vi "Fpga-MicroBlaze-Top.vi"() -> ()   [LabVIEW 2017]
uses:
  <vilib>/Platform/TimedLoop/XDataNode/timing_clust.ctl
  <vilib>/Platform/TimedLoop/XDataNode/nitl_modes.ctl
  <vilib>/Platform/TimedLoop/XDataNode/wakeup.ctl
  <vilib>/rvi/Emulation/niFpgaSctlEmulationGetInTimedLoop.vi
  <vilib>/rvi/Emulation/niFpgaEmulationReportErrorSimple.vi
  <vilib>/rvi/Emulation/niFpgaGetClockAttributes.vi
  <vilib>/rvi/Emulation/niFpgaCriticalErrorInLSC.vi
  <vilib>/rvi/eio/common/nirviEmuTemplateMethod_errors.vi
  <vilib>/rvi/interface/RandomDataEmulation/niFpgaRandomDataHandleErrors.vi
  <vilib>/Platform/TimedLoop/XDataNode/XDataNode.xnode
  <vilib>/eio/EIONode/EIONode.xnode
  <vilib>/rvi/DataTransferAndStorage/Container/XNode/niFpgaContainer.xnode
  <vilib>/rvi/interface/RandomDataEmulation/nirviRandomDataFpgaReadWriteTemplate.vi
  <vilib>/Platform/TimedLoop/XDataNode/XDNodeRunTimeDep.lvlib
panel:
  out "d_microblaze_i\\AXI_STR_TXD_1_tkeep":fxp<+,4,4>
  in  "d_microblaze_i\\AXI_STR_RXD_1_tkeep":fxp<+,4,4>
  out "d_microblaze_i\\AXI_STR_TXD_tkeep":fxp<+,4,4>
  in  "d_microblaze_i\\AXI_STR_RXD_tkeep":fxp<+,4,4>
  in  "d_microblaze_i\\reset_rtl":bool=TRUE
  out "HeartBeat X 2":i16
  in  "HeartBeat":i16
  out "AXI_STR_RXD_tready 1":bool
  out "tvalid 1":bool
  out "tdata 1":u32
  out "tlast 1":bool
  out "AXI_STR_RXD_tready_Count 1":u16
  out "tvalid_Count 1":u16
  out "tlast_Count 1":u16
  out "tdata_LastNonZero 1":u32
  out "AXI_STR_RXD_tready 2":bool
  out "tvalid 2":bool
  out "tdata 2":u32
  out "tlast 2":bool
  out "AXI_STR_RXD_tready_Count 2":u16
  out "tvalid_Count 2":u16
  out "tlast_Count 2":u16
  out "tdata_LastNonZero 2":u32
  in  "Interrupt #1":bool
  in  "Interrupt #0":bool
  out "GPIO #2 out":u32 format="%.0x"
  in  "GPIO #2 in":u32
  out "GPIO #1 out":u32 format="%.0x"
  in  "GPIO #1 in":u32
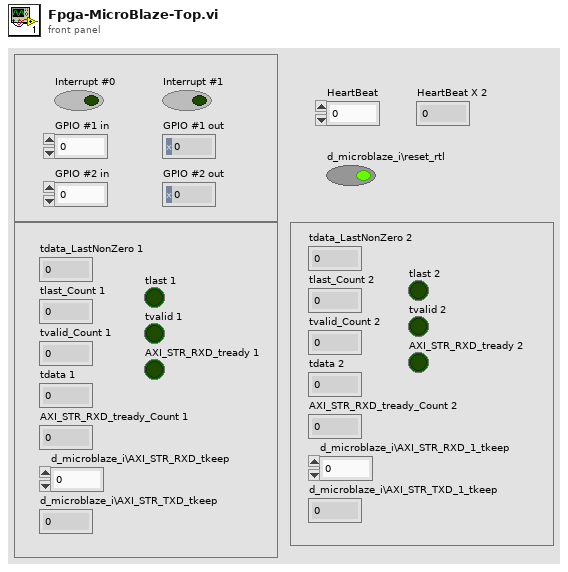
[diagram p1: front panel]
types:
  T1 = typedef "XDNodeRunTimeDep.lvlib/timing_clust.ctl" = cluster{"Expected End [f-1]":u64, "Actual End [f-1]":u64, "Finished Late? [f-1]":bool, "Expected End [i-1]":u64, "Actual End [i-1]":u64, "Finished Late? [i-1]":bool, "Expected Start [i]":u64, "Actual Start [i]":u64, "Expected Start [f]":u64, "Actual Start [f]":u64, "Source Name":string, "Structure Name":string, "Period":i64, "Deadline":i64, "Offset":i64, "Start":i64, "Priority":i32, "Timeout":i32, "Mode":T2, "Wakeup Reason":T3, "Error":errorcluster, "Source Type":string, "Secondary Source Type":string, "Global End Time":u64, "Global Start Time":u64, "Frame Duration":u64, "Iteration Duration":u64, "Assigned CPU":i32, "I/O Scan Engine Mode":u32}
  T2 = typedef "XDNodeRunTimeDep.lvlib/nitl_modes.ctl" = enum32{"No Change", "Process missed periods, maintain original phase", "Discard missed periods, maintain original phase", "Process missed periods, ignore original phase", "Discard missed periods, ignore original phase"}
  T3 = typedef "XDNodeRunTimeDep.lvlib/wakeup.ctl" = enum32{"Normal", "Aborted", "Asynchronous wakeup", "Timing source error", "Timed loop error", "Timeout"}
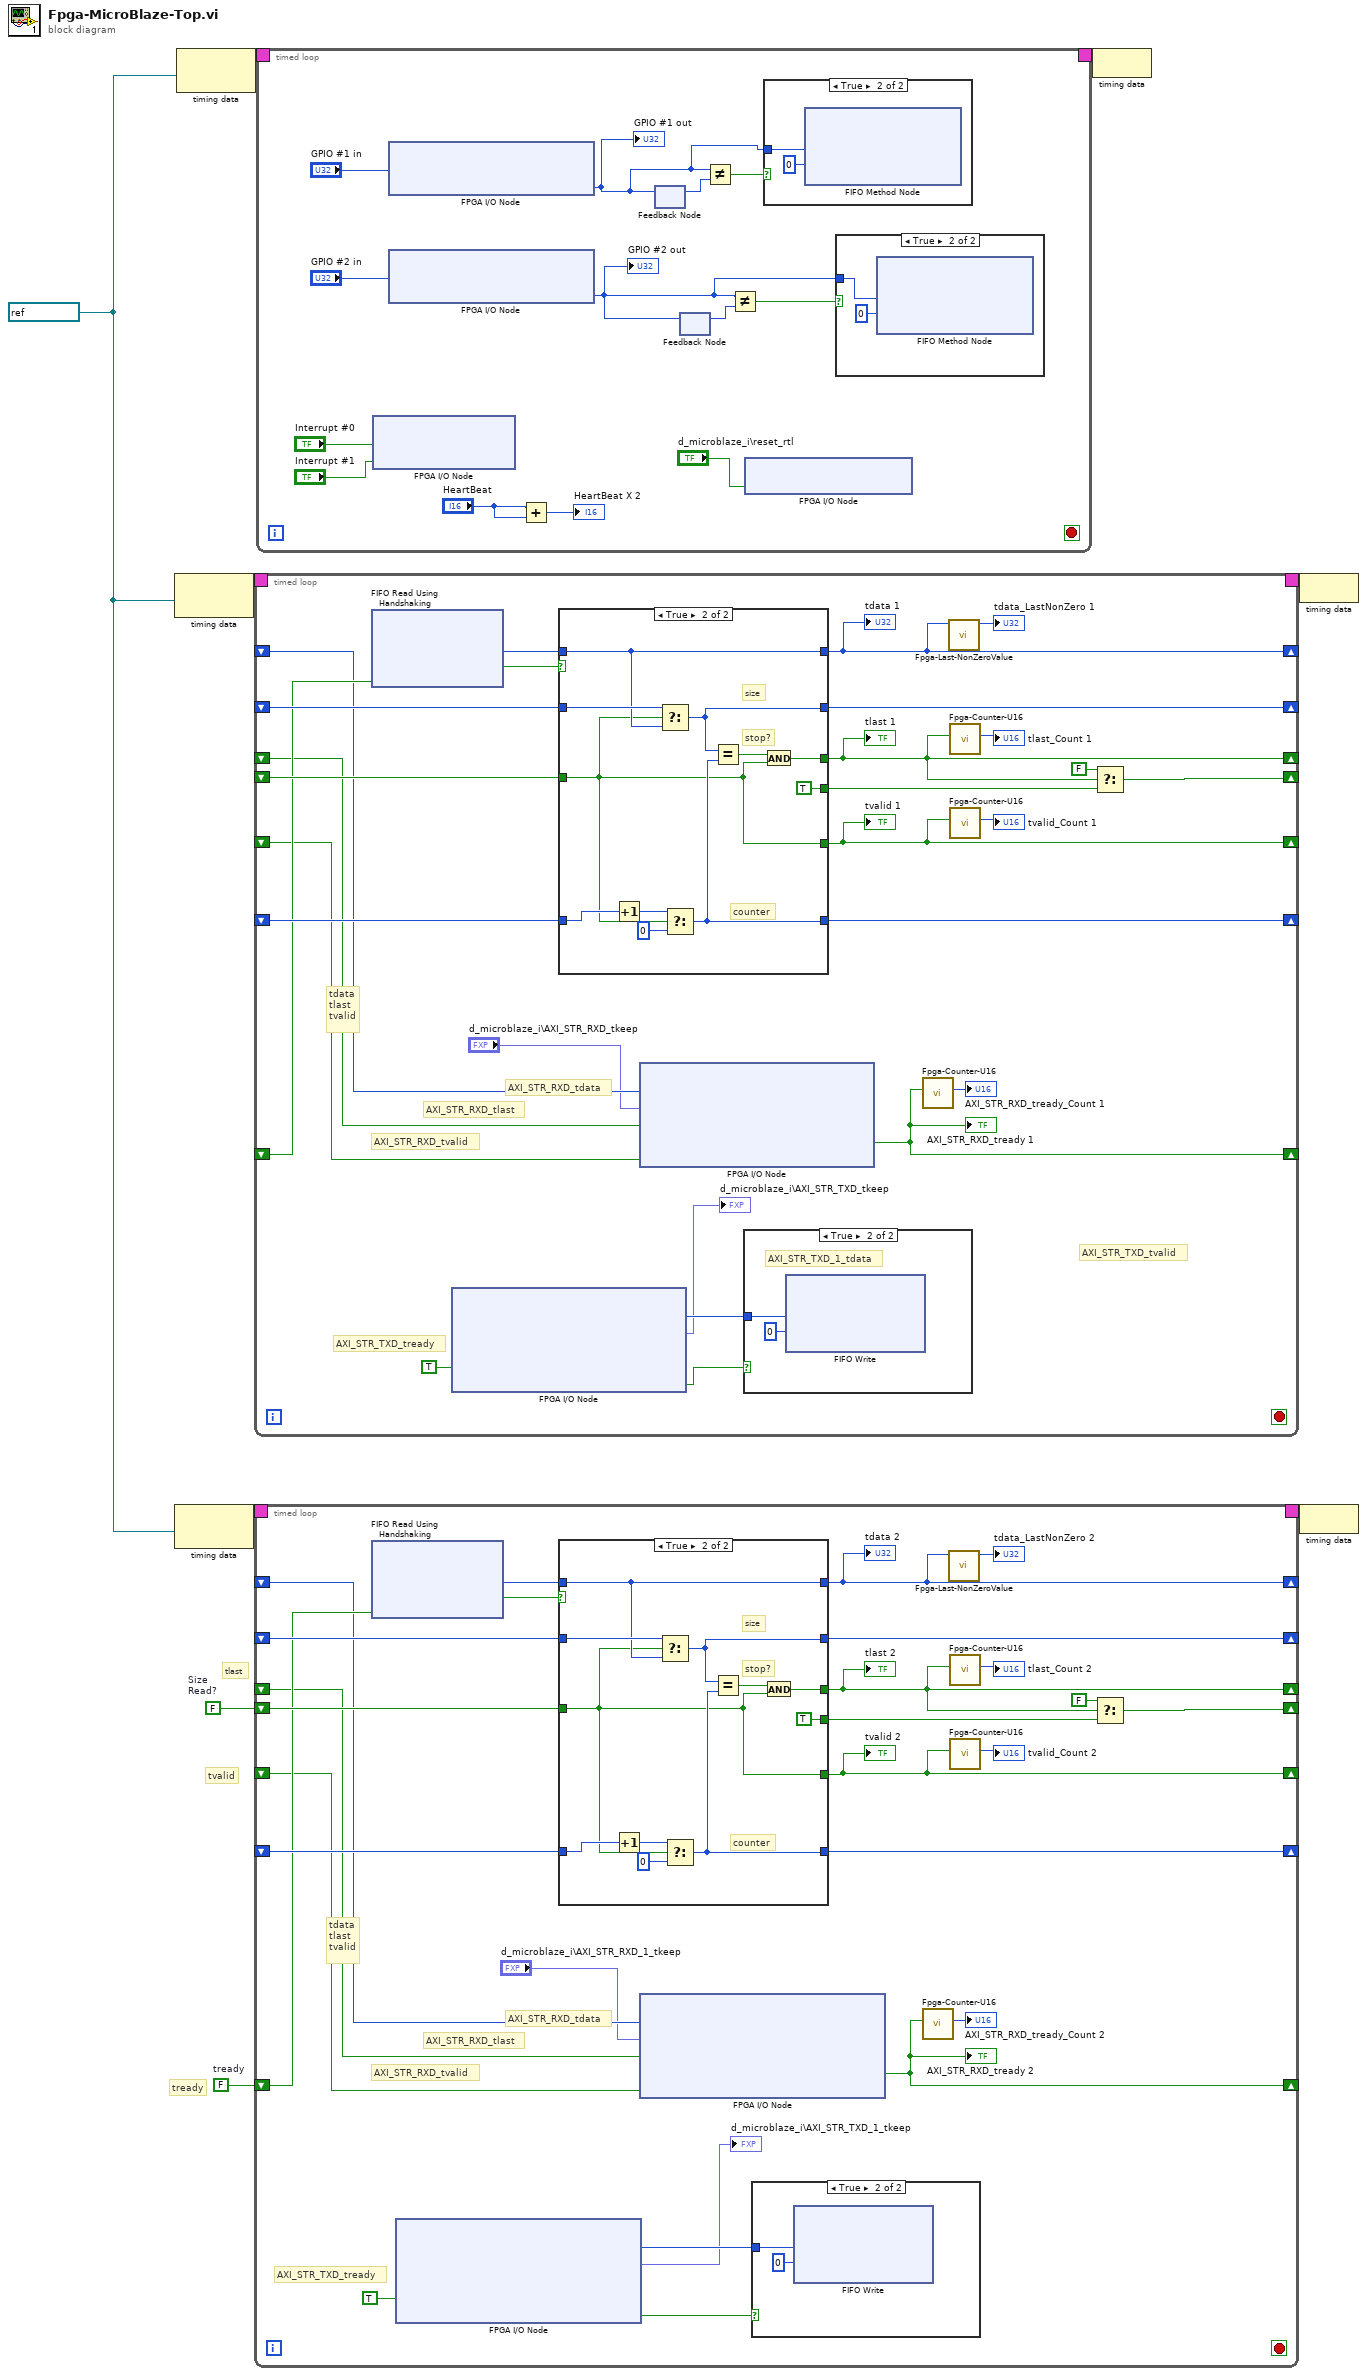
[diagram p0: block diagram]
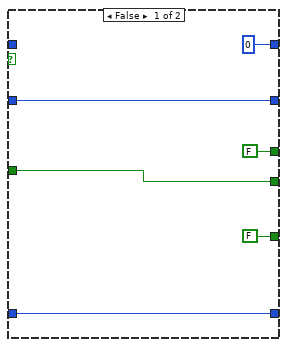
[diagram p3: hidden frame]
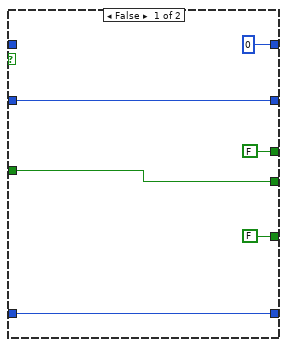
[diagram p5: hidden frame]
diagram:
  w4 = FALSE  # Size Read?
  w5 = FALSE  # tready
  w3 = refnum<k21> "100MHz" ("Source Name")
  # "tlast"
  # "tvalid"
  # "tready"
  n1 = node-c288(w3) -> (w2:T1)
  n2 = node-c288(w3) -> (w7:T1)
  n3 = node-c288(w3) -> (w9:T1)
  n4 = timed-loop {
    timing: w2 -> [_]
    timing-out: [_] -> w1
    shift-right: [w17] -> _
    shift-left: _ -> [w35]
    shift-right: [w32] -> _
    shift-left: _ -> [w34]
    shift-right: [w30] -> _
    shift-left: _ -> [w31]
    shift-right: [w13] -> _
    shift-left: _ -> [w23]
    shift-right: [w12] -> _
    shift-left: _ -> [w29]
    shift-right: [w27] -> _
    shift-left: _ -> [w25]
    shift-right: [w16] -> _
    shift-left: _ -> [w24]
    stop <- _ stop-if-true
    # "AXI_STR_TXD_tvalid"
    # "AXI_STR_TXD_tready"
    # "AXI_STR_RXD_tvalid"
    # "AXI_STR_RXD_tlast"
    # "AXI_STR_RXD_tdata"
    # "tdata\ntlast\ntvalid"
    n5 = xnode ("FIFO Read Using Handshaking")("Ready for Output"=w29) -> ("Element"=w33:u32, "Output Valid"=w36:bool)  [unwired: 1 in, 1 out]
    n6 = xnode "FPGA I/O Node"("d_microblaze_i\\AXI_STR_TXD_tready"=TRUE ("d_microblaze\\AXI_STR_TXD_tready")) -> ("d_microblaze_i\\AXI_STR_TXD_tdata"=w20:u32, "d_microblaze_i\\AXI_STR_TXD_tkeep"=→"d_microblaze_i\\AXI_STR_TXD_tkeep":fxp<+,4,4>, "d_microblaze_i\\AXI_STR_TXD_tvalid"=w21:bool)  [unwired: 5 in, 6 out]
    n7 = case shown="True" w36 {
      tunnel: w35 -> [w43 w45]
      tunnel: [w43 TRUE ("Size\nRead?")] -> w18
      tunnel: w34 -> [w44 w55]
      tunnel: w33 -> [_ w50]
      tunnel: [w44 w49] -> w32
      tunnel: w31 -> [w42 w54]
      tunnel: [w42 w48] -> w30
      tunnel: [FALSE ("Size\nRead?") w45] -> w13
      tunnel: [u32 0 ("Element") w50] -> w27
      tunnel: [FALSE w46] -> w16
      frame False {
      }
      frame True {
        # "stop?"
        # "size"
        # "counter"
        n8 = Increment(x=w54) -> (x+1=w52:u32)
        n9 = Select(t=w55, s=w45, f=w50) -> (s? t:f=w49:u32)
        n10 = Select(t=w52, s=w45, f=u32 0) -> (s? t:f=w48:u32)
        n11 = Equal?(x=w49, y=w48) -> (x = y?=w47:bool)
        n12 = And(x=w47, y=w45) -> (x .and. y?=w46:bool)
      }
    }
    "tvalid 1" <- w13
    "tdata 1" <- w27
    "tlast 1" <- w16
    n13 = xnode "FPGA I/O Node"("d_microblaze_i\\AXI_STR_RXD_tdata"=w25, "d_microblaze_i\\AXI_STR_RXD_tkeep"="d_microblaze_i\\AXI_STR_RXD_tkeep", "d_microblaze_i\\AXI_STR_RXD_tlast"=w24, "d_microblaze_i\\AXI_STR_RXD_tvalid"=w23) -> ("d_microblaze_i\\AXI_STR_RXD_tready"=w12:bool)  [unwired: 5 in, 5 out]
    "AXI_STR_RXD_tready 1" <- w12
    n14 = case shown="True" w21 {
      tunnel: w20 -> [_ w38]
      frame False {
      }
      frame True {
        # "AXI_STR_TXD_1_tdata"
        n15 = xnode ("FIFO Write")("Element"=w38, "Timeout"=0) -> ()  [unwired: 1 in, 2 out]
      }
    }
    n16 = call "Fpga-Counter-U16.vi"("d_mcs_i\\IO_BUS_read_strobe"=w12) -> ("Numeric"=→"AXI_STR_RXD_tready_Count 1":u16)  [unwired: 10 in]
    n17 = call "Fpga-Last-NonZeroValue.vi"("d_mcs_i\\IO_BUS_write_data in"=w27) -> ("d_mcs_i\\IO_BUS_write_data out"=→"tdata_LastNonZero 1":u32)  [unwired: 10 in]
    n18 = call "Fpga-Counter-U16.vi"("d_mcs_i\\IO_BUS_read_strobe"=w16) -> ("Numeric"=→"tlast_Count 1":u16)  [unwired: 10 in]
    n19 = call "Fpga-Counter-U16.vi"("d_mcs_i\\IO_BUS_read_strobe"=w13) -> ("Numeric"=→"tvalid_Count 1":u16)  [unwired: 10 in]
    n20 = Select(t=FALSE, s=w16, f=w18) -> (s? t:f=w17:bool)
  }
  n21 = timed-loop {
    timing: w7 -> [_]
    timing-out: [_] -> w6
    shift-right: [w65] -> _
    shift-left: w4 -> [w83]
    shift-right: [w80] -> _
    shift-left: _ -> [w82]
    shift-right: [w78] -> _
    shift-left: _ -> [w79]
    shift-right: [w61] -> _
    shift-left: _ -> [w71]
    shift-right: [w60] -> _
    shift-left: w5 -> [w77]
    shift-right: [w75] -> _
    shift-left: _ -> [w73]
    shift-right: [w64] -> _
    shift-left: _ -> [w72]
    stop <- _ stop-if-true
    # "AXI_STR_TXD_tready"
    # "AXI_STR_RXD_tvalid"
    # "AXI_STR_RXD_tlast"
    # "AXI_STR_RXD_tdata"
    # "tdata\ntlast\ntvalid"
    n22 = xnode ("FIFO Read Using Handshaking")("Ready for Output"=w77) -> ("Element"=w81:u32, "Output Valid"=w84:bool)  [unwired: 1 in, 1 out]
    n23 = xnode "FPGA I/O Node"("d_microblaze_i\\AXI_STR_TXD_1_tready"=TRUE ("d_microblaze\\AXI_STR_TXD_tready")) -> ("d_microblaze_i\\AXI_STR_TXD_1_tdata"=w68:u32, "d_microblaze_i\\AXI_STR_TXD_1_tkeep"=→"d_microblaze_i\\AXI_STR_TXD_1_tkeep":fxp<+,4,4>, "d_microblaze_i\\AXI_STR_TXD_1_tvalid"=w69:bool)  [unwired: 5 in, 6 out]
    n24 = case shown="True" w84 {
      tunnel: w83 -> [w91 w93]
      tunnel: [w91 TRUE ("Size\nRead?")] -> w66
      tunnel: w82 -> [w92 w103]
      tunnel: w81 -> [_ w98]
      tunnel: [w92 w97] -> w80
      tunnel: w79 -> [w90 w102]
      tunnel: [w90 w96] -> w78
      tunnel: [FALSE ("Size\nRead?") w93] -> w61
      tunnel: [u32 0 ("Element") w98] -> w75
      tunnel: [FALSE w94] -> w64
      frame False {
      }
      frame True {
        # "stop?"
        # "size"
        # "counter"
        n25 = Increment(x=w102) -> (x+1=w100:u32)
        n26 = Select(t=w103, s=w93, f=w98) -> (s? t:f=w97:u32)
        n27 = Select(t=w100, s=w93, f=u32 0) -> (s? t:f=w96:u32)
        n28 = Equal?(x=w97, y=w96) -> (x = y?=w95:bool)
        n29 = And(x=w95, y=w93) -> (x .and. y?=w94:bool)
      }
    }
    "tvalid 2" <- w61
    "tdata 2" <- w75
    "tlast 2" <- w64
    n30 = xnode "FPGA I/O Node"("d_microblaze_i\\AXI_STR_RXD_1_tdata"=w73, "d_microblaze_i\\AXI_STR_RXD_1_tkeep"="d_microblaze_i\\AXI_STR_RXD_1_tkeep", "d_microblaze_i\\AXI_STR_RXD_1_tlast"=w72, "d_microblaze_i\\AXI_STR_RXD_1_tvalid"=w71) -> ("d_microblaze_i\\AXI_STR_RXD_1_tready"=w60:bool)  [unwired: 5 in, 5 out]
    "AXI_STR_RXD_tready 2" <- w60
    n31 = case shown="True" w69 {
      tunnel: w68 -> [_ w86]
      frame False {
      }
      frame True {
        n32 = xnode ("FIFO Write")("Element"=w86, "Timeout"=0) -> ()  [unwired: 1 in, 2 out]
      }
    }
    n33 = call "Fpga-Counter-U16.vi"("d_mcs_i\\IO_BUS_read_strobe"=w60) -> ("Numeric"=→"AXI_STR_RXD_tready_Count 2":u16)  [unwired: 10 in]
    n34 = call "Fpga-Last-NonZeroValue.vi"("d_mcs_i\\IO_BUS_write_data in"=w75) -> ("d_mcs_i\\IO_BUS_write_data out"=→"tdata_LastNonZero 2":u32)  [unwired: 10 in]
    n35 = call "Fpga-Counter-U16.vi"("d_mcs_i\\IO_BUS_read_strobe"=w64) -> ("Numeric"=→"tlast_Count 2":u16)  [unwired: 10 in]
    n36 = call "Fpga-Counter-U16.vi"("d_mcs_i\\IO_BUS_read_strobe"=w61) -> ("Numeric"=→"tvalid_Count 2":u16)  [unwired: 10 in]
    n37 = Select(t=FALSE, s=w64, f=w66) -> (s? t:f=w65:bool)
  }
  n38 = timed-loop {
    timing: w9 -> [_]
    timing-out: [_] -> w8
    stop <- _ stop-if-true
    n39 = xnode "FPGA I/O Node"("d_microblaze_i\\In0"="Interrupt #0", "d_microblaze_i\\In1"="Interrupt #1") -> ()  [unwired: 2 in, 2 out]
    n40 = xnode "FPGA I/O Node"("d_microblaze_i\\gpio_rtl_tri_i"="GPIO #1 in") -> ("d_microblaze_i\\gpio_rtl_0_tri_o"=w106:u32)  [unwired: 2 in, 2 out]
    "GPIO #1 out" <- w106
    n41 = xnode "FPGA I/O Node"("d_microblaze_i\\gpio_rtl_1_tri_i"="GPIO #2 in") -> ("d_microblaze_i\\gpio_rtl_2_tri_o"=w108:u32)  [unwired: 2 in, 2 out]
    "GPIO #2 out" <- w108
    n42 = Add(x="HeartBeat", y="HeartBeat") -> (x+y=→"HeartBeat X 2":i16)
    n43 = feedback #1() -> (w110:u32)  [unwired: 1 in]
    n44 = feedback-in #1(w106) -> ()
    n45 = feedback #2() -> (w113:u32)  [unwired: 1 in]
    n46 = feedback-in #2(w108) -> ()
    n47 = Not Equal?(x=w106, y=w110) -> (x != y?=w107:bool)
    n48 = Not Equal?(x=w108, y=w113) -> (x != y?=w109:bool)
    n49 = xnode "FPGA I/O Node"("d_microblaze_i\\reset_rtl"="d_microblaze_i\\reset_rtl") -> ()  [unwired: 1 in, 1 out]
    n50 = case shown="True" w107 {
      tunnel: w106 -> [_ w120]
      frame False {
      }
      frame True {
        n51 = xnode ("FIFO Method Node")("Element"=w120, "Timeout"=0) -> ()  [unwired: 1 in, 2 out]
      }
    }
    n52 = case shown="True" w109 {
      tunnel: w108 -> [_ w122]
      frame False {
      }
      frame True {
        n53 = xnode ("FIFO Method Node")("Element"=w122, "Timeout"=0) -> ()  [unwired: 1 in, 2 out]
      }
    }
  }
  n54 = node-c288(w8) -> ()
  n55 = node-c288(w1) -> ()
  n56 = node-c288(w6) -> ()
